vi "Main.vi"() -> ()   [LabVIEW 2020, in "plugin_flodx_ph_probe.lvlib"]
doc: "pH Probe Plugin"
uses:
  plugin_flodx_ph_probe.lvlib
  plugin/process loops/Instrument Manager/loop/Instrument Loop State.ctl
  plugin/process loops/Instrument Manager/connection_info/Connection Info.ctl
  plugin/process loops/Instrument Manager/Instrument State.ctl
  plugin/process loops/UI Manager/Data Display Loop Data.ctl
  plugin/process loops/UI Manager/UI Data.ctl
  plugin/process loops/UI Manager/dialogs/settings/settings.ctl
  <userlib>/RxnRover/PluginCore/src/process loops/Acquisition/Acquisition Config.ctl
  plugin/process loops/Instrument Manager/Instrument Config.ctl
  <userlib>/RxnRover/PluginCore/src/process loops/Logging/loop/Logging Config.ctl
  <userlib>/RxnRover/PluginCore/src/process loops/Logging/log formats/Supported Log File Formats.ctl
  <userlib>/RxnRover/PluginCore/src/process loops/Logging/logger/Logging Start Mode.ctl
  <userlib>/RxnRover/PluginCore/src/process loops/Logging/logger/Logging Stop Mode.ctl
  plugin/process loops/System Control/System Control Data.ctl
  plugin/process loops/UI Manager/UI Display State.ctl
  56943c0d-d29c-4187-abe8-fcc35b9a4d89.vi
  aa3e49f4-ec9d-4bab-88e0-6a79f4e22ab8.vi
  <vilib>/Utility/error.llb/Error Cluster From Error Code.vi
  <vilib>/JDP Science/JSONtext/Variant to JSON Text.vi
  <vilib>/ErrorRing/Error Ring.xnode
  <vilib>/JDP Science/JSONtext/LVClass Serializer/JSONtext LVClass Serializer.lvclass
  <userlib>/RxnRover/PluginCore/src/support/Message Queue/Message Queue.lvlib
  plugin/plugin.lvlib
  <userlib>/RxnRover/PluginCore/src/process loops/Message Queues/Message Queues.lvlib
  <userlib>/RxnRover/PluginCore/src/support/User Event - Stop/User Event - Stop.lvlib
  plugin/process loops/Instrument Manager/Instrument Manager.lvlib
  <userlib>/RxnRover/PluginCore/src/process loops/Logging/Logging.lvlib
  <userlib>/RxnRover/PluginCore/src/process loops/Acquisition/Acquisition.lvlib
  <userlib>/RxnRover/PluginCore/src/process loops/Remote Connection Manager/Remote Connection Manager.lvlib
panel:
  in  "Restart":bool
  out "Comp. Temp(C)":sgl
  out "Address":u8
  in  "Open Calibrate Btn":bool
  out "Logging?":bool
  in  "Time Interval (sec)":i32=1200
  out "Data Graph":cluster{timestamp[], dbl[]}[](graph)
  in  "Open Settings Btn":bool
  in  "Toggle Logging":bool
  out "Measured pH":sgl format="%.2f pH"
  out "VISA resource":refnum<visa-resource-name>
  # "FloDx pH Probe"
  # "Configuration"
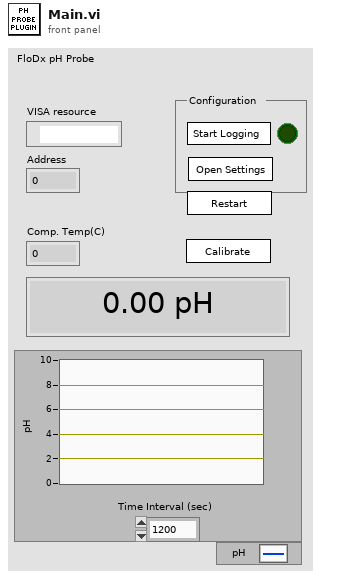
[diagram p1: front panel]
types:
  T1 = typedef "plugin_flodx_ph_probe.lvlib/plugin.lvlib/System Control Data.ctl" = cluster{"Example Value <Replace Me>":dbl, "Log Runs":bool, "Clone":bool}
  T2 = typedef "plugin_flodx_ph_probe.lvlib/plugin.lvlib/UI Data.ctl" = cluster{"UI Controls":cluster{"VISA Resource Ind":refnum<vi>, "Settings Btn":refnum<vi>, "Data Graph":refnum<vi>, "Logging Indicator":refnum<vi>, "Toggle Logging Btn":refnum<vi>, "Measured pH":refnum<vi>, "Temperature (C)":refnum<vi>, "Address":refnum<vi>, "Calibrate Btn":refnum<vi>}, "Plugin Settings":T3}
  T3 = typedef "plugin_flodx_ph_probe.lvlib/plugin.lvlib/settings.ctl" = cluster{"Acquisition Configuration":T4, "Instrument Configuration":T5, "Logging Configuration":T6, "Connection Info":T10}
  T4 = typedef "RxnRover_Plugin_Core.lvlib/Acquisition.lvlib/Acquisition Config.ctl" = cluster{"Query rate (sec)":dbl}
  T5 = typedef "plugin_flodx_ph_probe.lvlib/plugin.lvlib/Instrument Manager.lvlib/Instrument Config.ctl" = cluster{"Address":dbl, "Device":string, "Firmware Version":string}
  T6 = typedef "RxnRover_Plugin_Core.lvlib/Logging.lvlib/Logging Config.ctl" = cluster{"Log Directory":path, "Log File Format":T7, "Log File Name Prefix":string, "Logging Start Mode":T8, "Logging Stop Mode":T9, "Log Interval (Seconds)":dbl}
  T7 = typedef "RxnRover_Plugin_Core.lvlib/Logging.lvlib/Supported Log File Formats.ctl" = enum16{"Spreadsheet (CSV)"}
  T8 = typedef "RxnRover_Plugin_Core.lvlib/Logging.lvlib/Logging Start Mode.ctl" = enum16{"Manual Start", "Log While Running"}
  T9 = typedef "RxnRover_Plugin_Core.lvlib/Logging.lvlib/Logging Stop Mode.ctl" = enum16{"Log Continuously", "Log While Running"}
  T10 = typedef "plugin_flodx_ph_probe.lvlib/plugin.lvlib/Instrument Manager.lvlib/Connection Info.ctl" = cluster{"VISA Resource":refnum<visa-resource-name>, "Address":u8}
  T11 = typedef "plugin_flodx_ph_probe.lvlib/plugin.lvlib/Data Display Loop Data.ctl" = cluster{"Data Timestamps":timestamp[], "Data Values":dbl[], "Previous Run State":bool}
  T12 = typedef "plugin_flodx_ph_probe.lvlib/plugin.lvlib/Instrument Manager.lvlib/Instrument Loop State.ctl" = cluster{"Connection Info":T10, "Running":bool, "Running Since":timestamp, "Instrument State":T13}
  T13 = typedef "plugin_flodx_ph_probe.lvlib/plugin.lvlib/Instrument Manager.lvlib/Instrument State.ctl" = cluster{"pH":sgl, "Temperature (C)":sgl, "Device":string, "Firmware Version":string, "Error Status":bool, "Error Code":i32, "Error Source":string}
  T14 = typedef "RxnRover_Plugin_Core.lvlib/Message Queues.lvlib/All Message Queues.ctl" = cluster{"Acquisition":refnum<queue>, "Instrument":refnum<queue>, "Logging":refnum<queue>, "Remote":refnum<queue>, "System Control":refnum<queue>, "UI":refnum<queue>}
  T15 = typedef "plugin_flodx_ph_probe.lvlib/plugin.lvlib/UI Display State.ctl" = enum16{"Shown", "Hidden"}
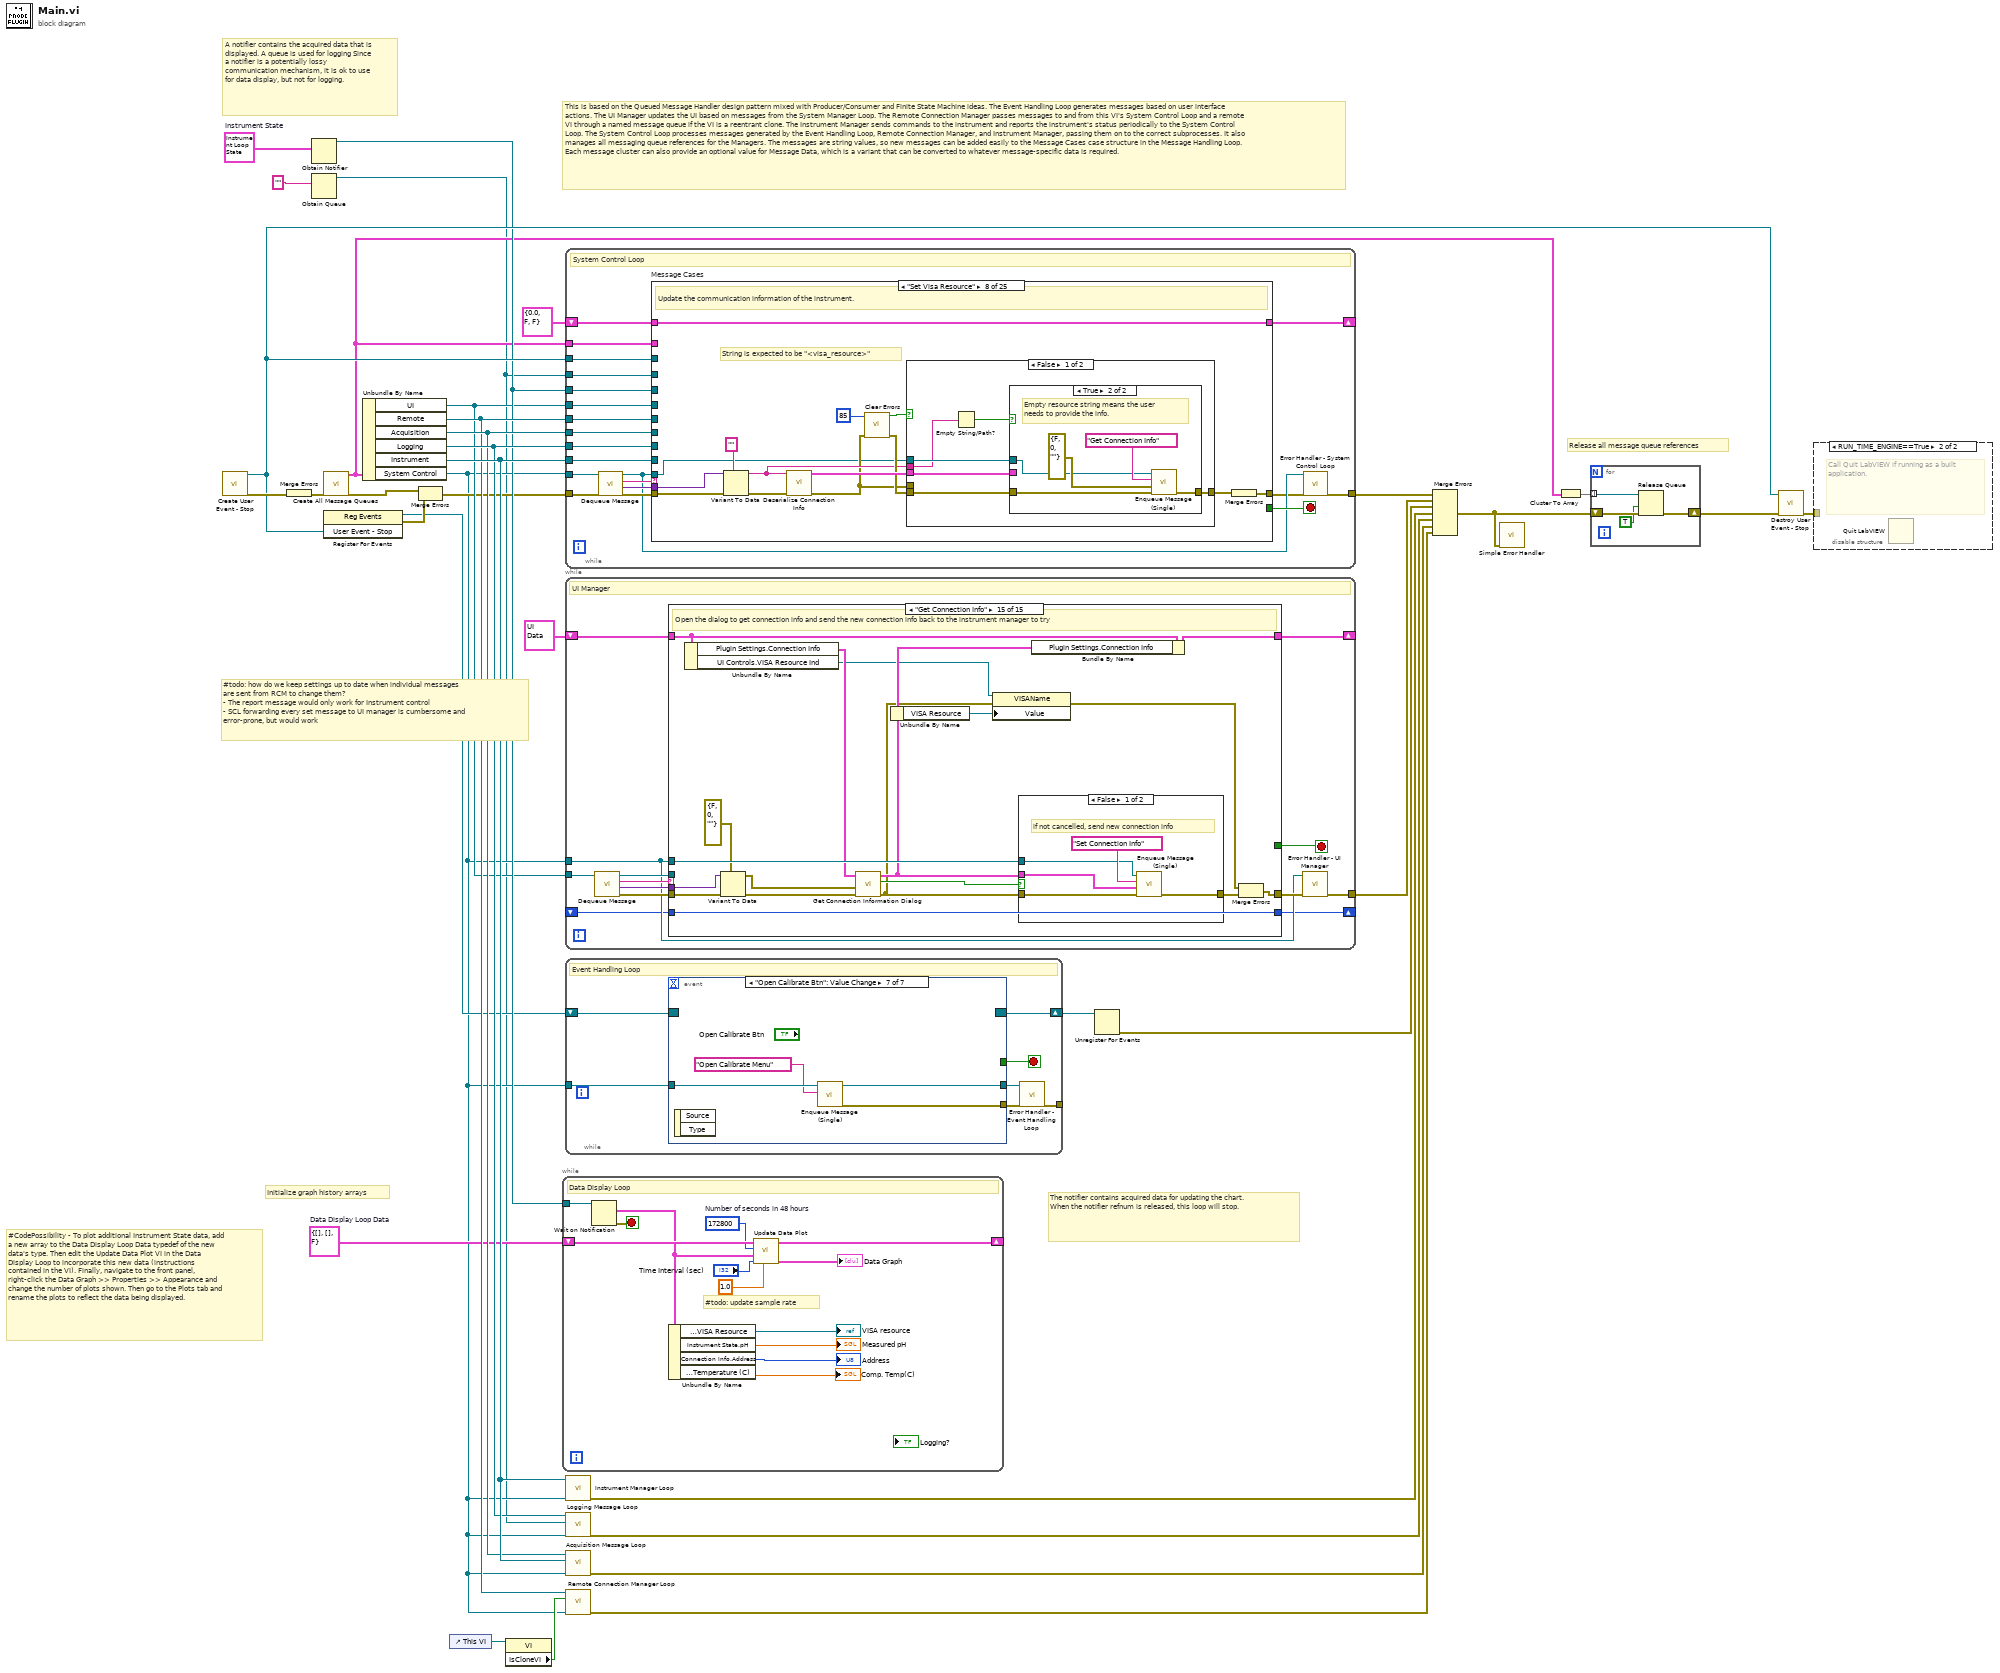
[diagram p0: block diagram]
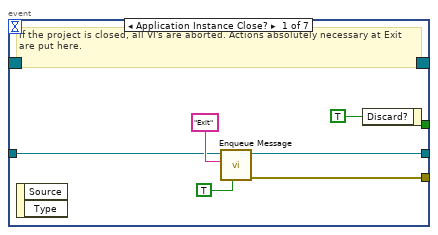
[diagram p2: hidden frame]
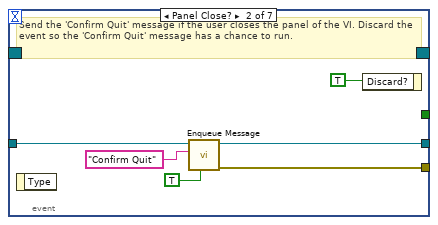
[diagram p3: hidden frame]
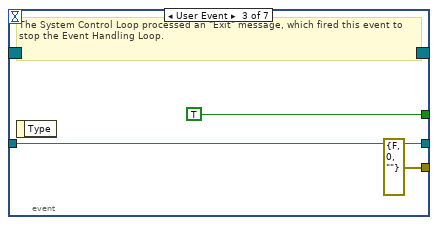
[diagram p4: hidden frame]
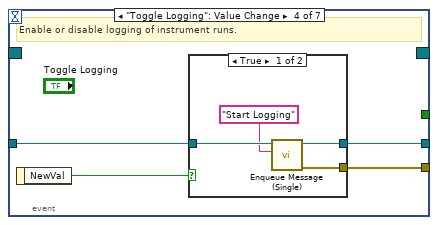
[diagram p5: hidden frame]
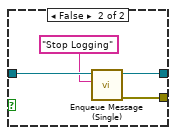
[diagram p6: hidden frame]
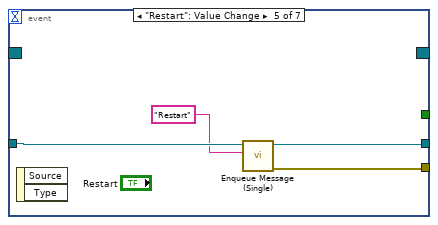
[diagram p7: hidden frame]
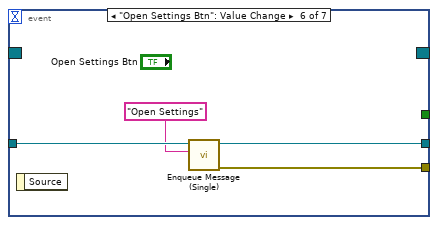
[diagram p8: hidden frame]
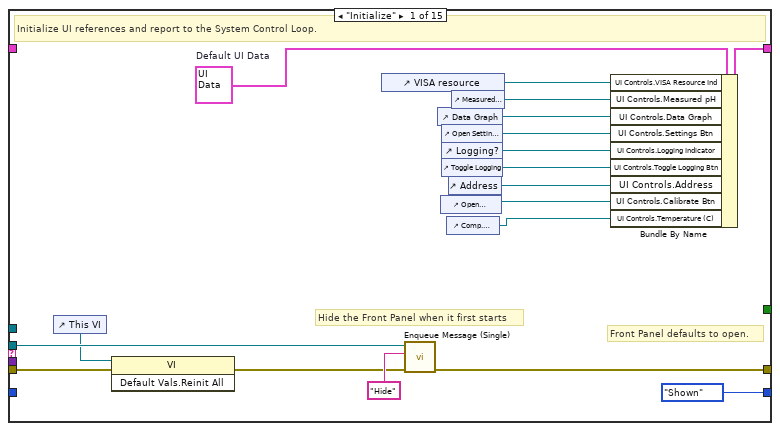
[diagram p9: hidden frame]
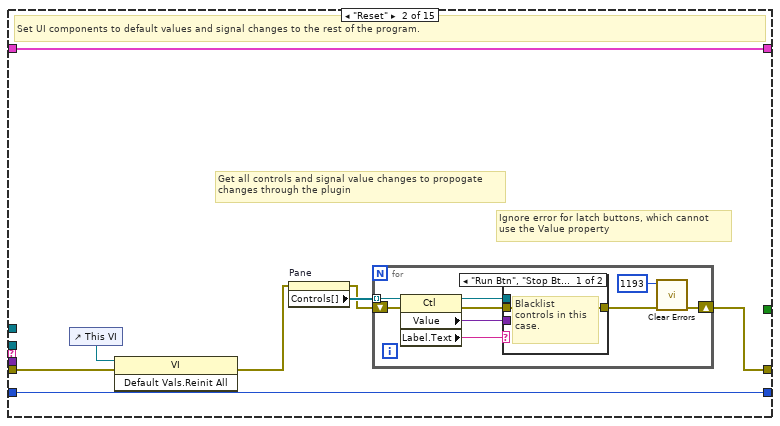
[diagram p10: hidden frame]
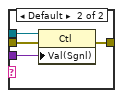
[diagram p11: hidden frame]
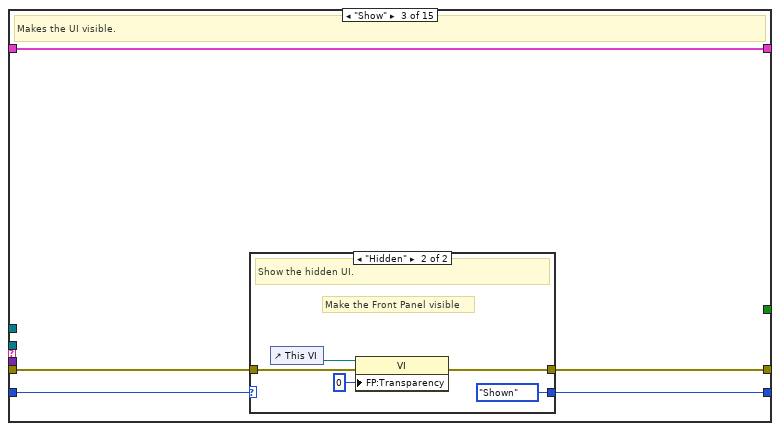
[diagram p12: hidden frame]
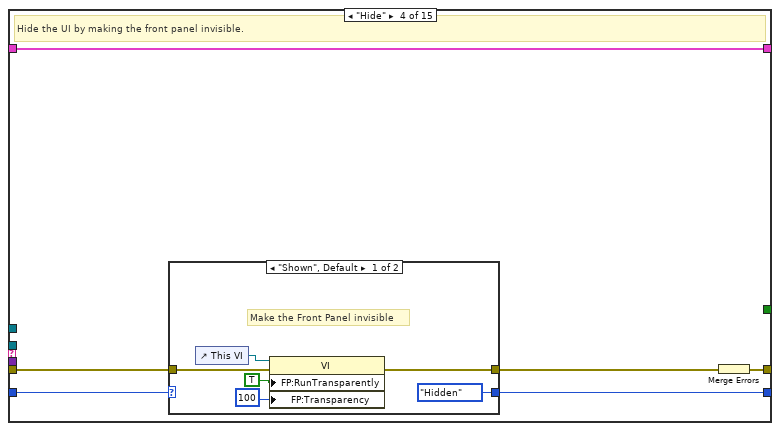
[diagram p14: hidden frame]
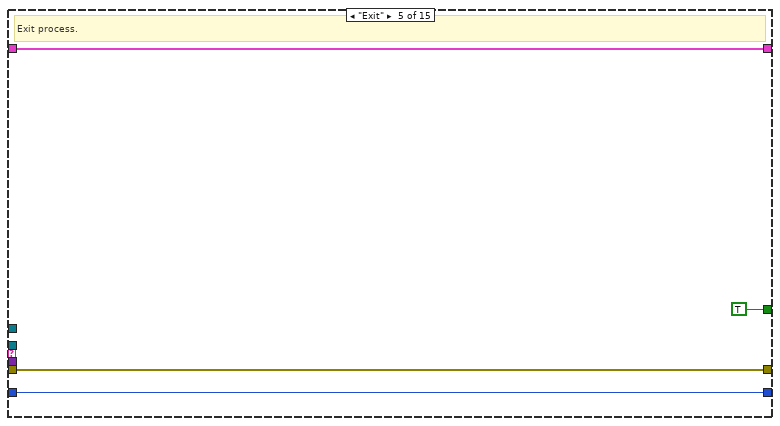
[diagram p16: hidden frame]
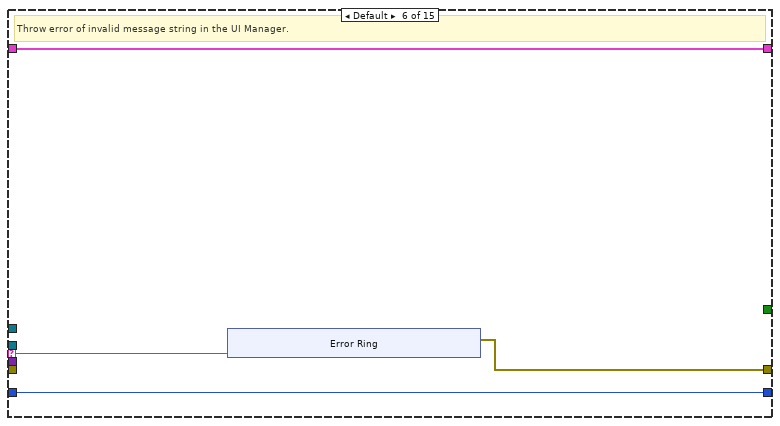
[diagram p17: hidden frame]
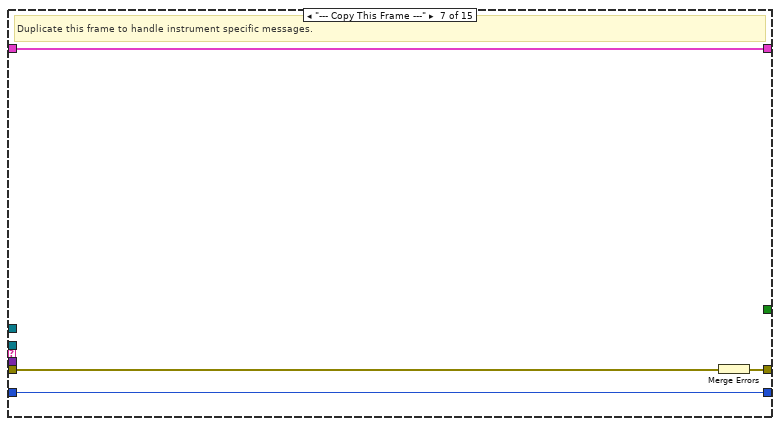
[diagram p18: hidden frame]
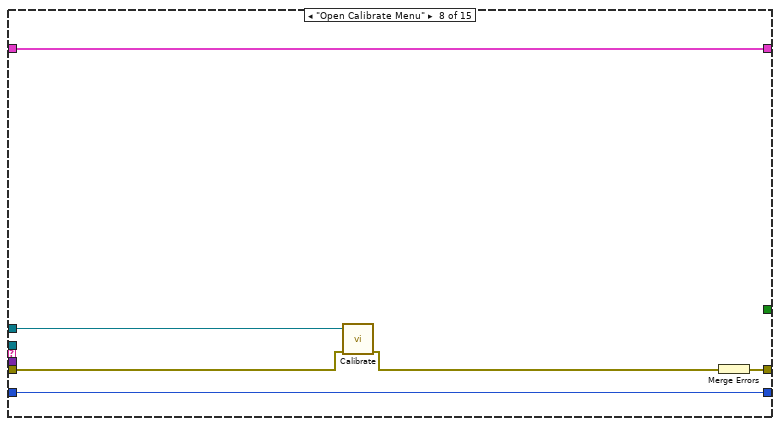
[diagram p19: hidden frame]
diagram:
  w9 = T11 {"Data Timestamps"=[], "Data Values"=[], "Previous Run State"=FALSE}  # Data Display Loop Data
  w12 = T12 {"Connection Info"={"VISA Resource"="", "Address"=0}, "Running"=FALSE, "Running Since"=timestamp(0 s since 1904-01-01), "Instrument State"={"pH"=0.0, "Temperature (C)"=0.0, "Device"="", "Firmware Version"="", "Error Status"=FALSE, "Error Code"=0, "Error Source"=""}}  # Instrument State
  # "#todo: how do we keep settings up to date when individual messages\nare sent from RCM to change them?\n- The report message would only work for Instrument control\n- SCL forwarding every set message to UI manager is cumbersome and\nerror-prone, but would work"
  # "#CodePossibility - To plot additional Instrument State data, add a new array to the Data Display Loop Data typedef of the new data's type. Then edit the Update Data Plot VI in the Data Display Loop to incorporate this new data (instructions contained in the VI). Finally, navigate to the front panel, right-click the Data Graph >> Properties >> Appearance and change the number of plots shown. Then go to the Plots tab and rename the plots to reflect the data being displayed."
  # "Initialize graph history arrays"
  # "A notifier contains the acquired data that is displayed. A queue is used for logging Since a notifier is a potentially lossy communication mechanism, it is ok to use for data display, but not for logging."
  # "The notifier contains acquired data for updating the chart. When the notifier refnum is released, this loop will stop."
  # "Release all message queue references"
  # "This is based on the Queued Message Handler design pattern mixed with Producer/Consumer and Finite State Machine ideas. The Event Handling Loop generates messages based on user interface actions. The UI Manager updates the UI based on messages from the System Manager Loop. The Remote Connection Manager passes messages to and from this VI's System Control Loop and a remote VI through a named message queue if the VI is a reentrant clone. The Instrument Manager sends commands to the instrument and reports the instrument's status periodically to the System Control Loop. The System Control Loop processes messages generated by the Event Handling Loop, Remote Connection Manager, and Instrument Manager, passing them on to the correct subprocesses. It also manages all messaging queue references for the Managers. The messages are string values, so new messages can be added easily to the Message Cases case structure in the Message Handling Loop.  Each message cluster can also provide an optional value for Message Data, which is a variant that can be converted to whatever message-specific data is required."
  n1 = call <userlib>:"Create User Event - Stop.vi"() -> ("error out"=w29:errorcluster, "User Event - Stop"=w25:refnum<user-event>)  [unwired: 10 in]
  n2 = Merge Errors(w29) -> (w28:errorcluster)
  n3 = Obtain Notifier(notification data type=w12) -> (notifier out=w13:refnum<notifier>)  [unwired: 3 in, 2 out]
  n4 = Obtain Queue(element data type="" ("<JSON>")) -> (queue out=w1:refnum<queue>)  [unwired: 4 in, 2 out]
  n5 = call <userlib>:"Create All Message Queues.vi"("error in (no error)"=w28) -> ("error out"=w31:errorcluster, "Message Queues out"=w7:T14)  [unwired: 9 in]
  n6 = register-events(w25) -> (reference out=w10:refnum<event-registration>, error out=w17:errorcluster)  [unwired: 2 in]
  n7 = Unbundle By Name(w7) -> ("UI"=w11:refnum<queue>, "Remote"=w32:refnum<queue>, "Acquisition"=w33:refnum<queue>, "Logging"=w34:refnum<queue>, "Instrument"=w35:refnum<queue>, "System Control"=w4:refnum<queue>)
  n8 = Merge Errors(w31, w17) -> (w5:errorcluster)
  n9 = control-ref of="This VI"() -> (w24:refnum<vi>)
  n10 = property class="VI"(reference=w24) -> ("IsCloneVI"=w23:bool)  [unwired: 1 in, 2 out]
  n11 = while "Data Display Loop" {
    tunnel: w13 -> [w48]
    shift-right: [w45] -> _
    shift-left: w9 -> [w46]
    stop <- w43 stop-if-true
    w40 = 172800  # Number of seconds in 48 hours
    # "#todo: update sample rate"
    # "Data Display Loop"
    n12 = Wait on Notification(notifier=w48) -> (notification=w38:T12, error out=w43:errorcluster)  [unwired: 3 in, 2 out]
    n13 = Unbundle By Name(w38) -> ("Connection Info.VISA Resource"=→"VISA resource":refnum<visa-resource-name>, "Instrument State.pH"=→"Measured pH":sgl, "Connection Info.Address"=→"Address":u8, "Instrument State.Temperature (C)"=→"Comp. Temp(C)":sgl)
    n14 = call "Update Data Plot.vi"("Sample Rate (sec/sample)"=1.0, "Time interval (s)"="Time Interval (sec)", "Instrument State"=w38, "History length (-1; unlimited)"=w40, "Graph History Arrays in"=w46) -> ("Updated Plot History"=→"Data Graph":cluster{timestamp[], dbl[]}[], "Graph History Arrays out"=w45:T11)  [unwired: 5 in]
  }
  n15 = while {
    tunnel: w11 -> [w61]
    tunnel: w4 -> [w52]
    tunnel: [w53] -> w22
    shift-right: [w56] -> _
    shift-left: T2 {"UI Controls"={"VISA Resource Ind"=refnum, "Settings Btn"=refnum, "Data Graph"=refnum, "Logging Indicator"=refnum, "Toggle Logging Btn"=refnum, "Measured pH"=refnum, "Temperature (C)"=refnum, "Address"=refnum, "Calibrate Btn"=refnum}, "Plugin Settings"={"Acquisition Configuration"={"Query rate (sec)"=0.0}, "Instrument Configuration"={"Address"=0.0, "Device"="", "Firmware Version"=""}, "Logging Configuration"={"Log Directory"=path "", "Log File Format"=enum."Spreadsheet (CSV)", "Log File Name Prefix"="", "Logging Start Mode"=enum."Manual Start", "Logging Stop Mode"=enum."Log Continuously", "Log Interval (Seconds)"=0.001}, "Connection Info"={"VISA Resource"="", "Address"=0}}} ("Default UI Data") -> [w55]
    shift-right: [w50] -> _
    shift-left: _ -> [w49]
    stop <- w51 stop-if-true
    # "UI Manager"
    n16 = call <userlib>:"Dequeue Message.vi"("Message Queue"=w61) -> ("error out"=w59:errorcluster, "Message Data"=w57:variant, "Message"=w58:string, "dup Message Queue"=w60:refnum<queue>)  [unwired: 7 in]
    n17 = case shown="\"Get Connection Info\"" w58 {
      selector: w58 -> [_ _ _ _ _ w135 _ _ _ _ _ _ _ w209 _]
      tunnel: w60 -> [w76 _ _ _ _ _ _ _ _ _ _ _ _ _ _]
      tunnel: w59 -> [w70 w83 w105 w117 w131 _ w144 w148 w153 w156 w162 w171 w186 w208 w251]
      tunnel: w57 -> [_ _ _ _ _ _ _ _ _ _ _ _ _ w205 w241]
      tunnel: w52 -> [_ _ _ _ _ _ _ w149 _ _ _ _ w177 _ w246]
      tunnel: [w71 w82 w104 w118 w131 w134 w145 w151 w153 w156 w167 w176 w187 w204 w252] -> w54
      tunnel: [w78 w80 w106 w119 w130 w133 w146 w152 w154 w157 w165 w174 w183 w206 w248] -> w56
      tunnel: w55 -> [_ w80 w106 w119 w130 w133 w146 w152 w154 w157 w165 w174 w184 w203 w249]
      tunnel: [_ _ _ _ TRUE _ _ _ _ _ _ _ _ _ _] -> w51
      tunnel: w49 -> [_ w81 w103 w115 w128 w132 w143 w150 w155 w158 w166 w175 w185 w211 w250]
      tunnel: [UI_Display_State."Shown" ("UI Display State") w81 w102 w114 w128 w132 w143 w150 w155 w158 w166 w175 w185 w211 w250] -> w50
      frame "Initialize" {
        w79 = T2 {"UI Controls"={"VISA Resource Ind"=refnum, "Settings Btn"=refnum, "Data Graph"=refnum, "Logging Indicator"=refnum, "Toggle Logging Btn"=refnum, "Measured pH"=refnum, "Temperature (C)"=refnum, "Address"=refnum, "Calibrate Btn"=refnum}, "Plugin Settings"={"Acquisition Configuration"={"Query rate (sec)"=0.0}, "Instrument Configuration"={"Address"=0.0, "Device"="", "Firmware Version"=""}, "Logging Configuration"={"Log Directory"=path "", "Log File Format"=enum."Spreadsheet (CSV)", "Log File Name Prefix"="", "Logging Start Mode"=enum."Manual Start", "Logging Stop Mode"=enum."Log Continuously", "Log Interval (Seconds)"=0.001}, "Connection Info"={"VISA Resource"="", "Address"=0}}}  # Default UI Data
        # "Front Panel defaults to open."
        # "Hide the Front Panel when it first starts"
        # "Initialize UI references and report to the System Control Loop."
        n18 = control-ref of="This VI"() -> (w72:refnum<vi>)
        n19 = invoke class="VI" method="Default Vals.Reinit All"(reference=w72, error in=w70) -> (error out=w69:errorcluster)  [unwired: 1 in, 2 out]
        n20 = control-ref of="VISA resource"() -> (w77:refnum<vi>)
        n21 = call <userlib>:"Enqueue Message (Single).vi"("error in (no error)"=w69, "Message"="Hide", "Message Queue"=w76) -> ("error out"=w71:errorcluster)  [unwired: 7 in, 1 out]
        n22 = control-ref of="Data Graph"() -> (w65:refnum<vi>)
        n23 = control-ref of="Open Calibrate Btn"() -> (w63:refnum<vi>)
        n24 = control-ref of="Open Settings Btn"() -> (w73:refnum<vi>)
        n25 = control-ref of="Logging?"() -> (w68:refnum<vi>)
        n26 = control-ref of="Toggle Logging"() -> (w67:refnum<vi>)
        n27 = control-ref of="Comp. Temp(C)"() -> (w62:refnum<vi>)
        n28 = control-ref of="Address"() -> (w64:refnum<vi>)
        n29 = control-ref of="Measured pH"() -> (w66:refnum<vi>)
        n30 = Bundle By Name(cluster=w79, "UI Controls.VISA Resource Ind"=w77, "UI Controls.Measured pH"=w66, "UI Controls.Data Graph"=w65, "UI Controls.Settings Btn"=w73, "UI Controls.Logging Indicator"=w68, "UI Controls.Toggle Logging Btn"=w67, "UI Controls.Address"=w64, "UI Controls.Calibrate Btn"=w63, "UI Controls.Temperature (C)"=w62) -> (w78:T2)
      }
      frame "Reset" {
        # "Ignore error for latch buttons, which cannot\nuse the Value property"
        # "Get all controls and signal value changes to propogate\nchanges through the plugin"
        # "Set UI components to default values and signal changes to the rest of the program."
        n31 = control-ref of="This VI"() -> (w87:refnum<vi>)
        n32 = invoke class="VI" method="Default Vals.Reinit All"(reference=w87, error in=w83) -> (error out=w84:errorcluster)  [unwired: 1 in, 2 out]
        n33 = property on="Pane" class="Pane"(error in=w84) -> (error out=w85:errorcluster, "Controls[]"=w86:refnum<vi>[])  [unwired: 1 in, 1 out]
        n34 = for {
          tunnel: w86 -> [w96] mode=indexing
          shift-right: [w90] -> w82
          shift-left: w85 -> [w95]
          n35 = property class="Ctl"(reference=w96, error in=w95) -> (reference out=w94:refnum<vi>, error out=w93:errorcluster, "Value"=w92:variant, "Label.Text"=w88:string)
          n36 = case shown="\"Run Btn\", \"Stop Btn\"" w88 {
            tunnel: w94 -> [_ w101]
            tunnel: w93 -> [w97 w100]
            tunnel: w92 -> [_ w99]
            tunnel: [w97 w98] -> w91
            frame "Run Btn", "Stop Btn" {
              # "Blacklist controls in this case."
            }
            frame Default {
              n37 = property class="Ctl"(reference=w101, error in=w100, "Val(Sgnl)"=w99) -> (error out=w98:errorcluster)  [unwired: 1 out]
            }
          }
          n38 = call <vilib>:"Clear Errors.vi"("error in (no error)"=w91, "specific error code to clear (0: all)"=1193) -> ("error out"=w90:errorcluster)  [unwired: 4 in, 1 out]
        }
      }
      frame "Show" {
        # "Makes the UI visible."
        n39 = case shown="\"Hidden\"" w103 {
          selector: w103 -> [w108 _]
          tunnel: w105 -> [w107 w113]
          tunnel: [w107 w111] -> w104
          tunnel: [w108 UI_Display_State."Shown" ("UI Display State")] -> w102
          frame "Shown", Default {
            # "Do nothing if UI is already shown."
          }
          frame "Hidden" {
            # "Make the Front Panel visible"
            # "Show the hidden UI."
            n40 = control-ref of="This VI"() -> (w112:refnum<vi>)
            n41 = property class="VI"(reference=w112, error in=w113, "FP:Transparency"=u8 0 ("Front Panel Window:Transparency")) -> (error out=w111:errorcluster)  [unwired: 1 out]
          }
        }
      }
      frame "Hide" {
        # "Hide the UI by making the front panel invisible."
        n42 = case shown="\"Shown\", Default" w115 {
          selector: w115 -> [_ w127]
          tunnel: w117 -> [w122 w126]
          tunnel: [w121 w126] -> w116
          tunnel: [UI_Display_State."Hidden" ("UI Display State") w127] -> w114
          frame "Shown", Default {
            # "Make the Front Panel invisible"
            n43 = control-ref of="This VI"() -> (w125:refnum<vi>)
            n44 = property class="VI"(reference=w125, error in=w122, "FP:RunTransparently"=TRUE ("Front Panel Window:Run VI Transparently"), "FP:Transparency"=u8 100 ("Front Panel Window:Transparency")) -> (error out=w121:errorcluster)  [unwired: 1 out]
          }
          frame "Hidden" {
          }
        }
        n45 = Merge Errors(w116) -> (w118:errorcluster)
      }
      frame "Exit" {
        # "Exit process."
      }
      frame Default {
        # "Throw error of invalid message string in the UI Manager."
        n46 = xnode "Error Ring"("parameter 0"=w135) -> ("error out"=w134:errorcluster)
      }
      frame "--- Copy This Frame ---" {
        # "Duplicate this frame to handle instrument specific messages."
        n47 = Merge Errors(w144) -> (w145:errorcluster)
      }
      frame "Open Calibrate Menu" {
        n48 = call "Calibrate.vi"("error in (no error)"=w148, "Message Queue"=w149) -> ("error out"=w147:errorcluster)  [unwired: 9 in]
        n49 = Merge Errors(w147) -> (w151:errorcluster)
      }
      frame "Instrument Started" {
        # "The instrument started. Ensure that the UI reflects this."
      }
      frame "Instrument Stopped" {
        # "The instrument stopped. Ensure that the UI reflects this."
      }
      frame "Logging Started" {
        w159 = TRUE  # Logging is on
        # "Indicate that logging started."
        n50 = Unbundle By Name(w165) -> ("UI Controls.Logging Indicator"=w164:refnum<vi>, "UI Controls.Toggle Logging Btn"=w163:refnum<vi>)
        n51 = property class="Bool (strict)"(reference=w164, error in=w162, "Value"=w159) -> (error out=w161:errorcluster)  [unwired: 1 out]
        n52 = property class="Bool"(reference=w163, error in=w162, "Value"=w159) -> (error out=w160:errorcluster)  [unwired: 1 out]
        n53 = Merge Errors(w161, w160) -> (w167:errorcluster)
      }
      frame "Logging Stopped" {
        w168 = FALSE  # Logging is off
        # "Indicate that logging stopped."
        n54 = Unbundle By Name(w174) -> ("UI Controls.Logging Indicator"=w173:refnum<vi>, "UI Controls.Toggle Logging Btn"=w172:refnum<vi>)
        n55 = property class="Bool (strict)"(reference=w173, error in=w171, "Value"=w168) -> (error out=w170:errorcluster)  [unwired: 1 out]
        n56 = property class="Bool"(reference=w172, error in=w171, "Value"=w168) -> (error out=w169:errorcluster)  [unwired: 1 out]
        n57 = Merge Errors(w170, w169) -> (w176:errorcluster)
      }
      frame "Open Settings" {
        # "Open the settings dialog and send new settings to other loops"
        n58 = Unbundle By Name(w184) -> ("Plugin Settings"=w182:T3)
        n59 = call "Settings Dialog.vi"("error in (no error)"=w186, "System Control Queue"=w177, "Plugin Settings"=w182) -> ("error out"=w181:errorcluster, "Cancelled?"=w179:bool, "Plugin Settings out"=w178:T3)  [unwired: 6 in]
        n60 = case shown="False" w179 {
          tunnel: w181 -> [w193 w201]
          tunnel: [w200 w201] -> w180
          tunnel: w178 -> [w195 _]
          tunnel: w177 -> [w194 _]
          frame False {
            # "Settings dialog was not cancelled, send new settings"
            n61 = Unbundle By Name(w195) -> ("Acquisition Configuration"=w198:T4)
            n62 = Unbundle By Name(w195) -> ("Instrument Configuration"=w196:T5)
            n63 = Unbundle By Name(w195) -> ("Logging Configuration"=w191:T6)
            n64 = call <userlib>:"Enqueue Message (Single).vi"("error in (no error)"=w193, "Message Data"=w198, "Message"="New Acquisition Config", "Message Queue"=w194) -> ("error out"=w188:errorcluster)  [unwired: 6 in, 1 out]
            n65 = call <userlib>:"Enqueue Message (Single).vi"("error in (no error)"=w193, "Message Data"=w196, "Message"="New Instrument Config", "Message Queue"=w194) -> ("error out"=w189:errorcluster)  [unwired: 6 in, 1 out]
            n66 = call <userlib>:"Enqueue Message (Single).vi"("error in (no error)"=w193, "Message Data"=w191, "Message"="New Logging Config", "Message Queue"=w194) -> ("error out"=w190:errorcluster)  [unwired: 6 in, 1 out]
            n67 = Merge Errors(w188, w189, w190) -> (w200:errorcluster)
          }
          frame True {
            # "The settings dialog was cancelled, don't send anything"
          }
        }
        n68 = Bundle By Name(cluster=w184, "Plugin Settings"=w178) -> (w183:T2)
        n69 = Merge Errors(w180) -> (w187:errorcluster)
      }
      frame "Acquisition Config", "Instrument Config", "Logging Config" {
        # "Store the settings provided by another loop to display to the user"
        n70 = Scan From String(format string="%s Config", input string=w209, error in=w208) -> (error out=w202:errorcluster, output 1=w207:string)  [unwired: 2 in, 2 out]
        n71 = case shown="\"Acquisition\"" w207 {
          tunnel: w203 -> [w213 w220 w227 w234]
          tunnel: [w213 w219 w226 w233] -> w206
          tunnel: w205 -> [_ w218 w225 w231]
          tunnel: w202 -> [w212 w217 w224 w230]
          tunnel: [w212 w216 w221 w229] -> w204
          frame Default {
            # "I don't know how we would get here, but do nothing\nif an invalid string is given."
          }
          frame "Acquisition" {
            n72 = Variant To Data(error in=w217, type=T4 {"Query rate (sec)"=1.0} ("Acquisition Configuration"), Variant=w218) -> (data=w215:T4, error out=w216:errorcluster)
            n73 = Bundle By Name(cluster=w220, "Plugin Settings.Acquisition Configuration"=w215) -> (w219:T2)
          }
          frame "Instrument" {
            n74 = Variant To Data(error in=w224, type=T5 {"Address"=0.0, "Device"="", "Firmware Version"=""} ("Instrument Configuration"), Variant=w225) -> (data=w222:T5, error out=w221:errorcluster)
            n75 = Bundle By Name(cluster=w227, "Plugin Settings.Instrument Configuration"=w222) -> (w226:T2)
          }
          frame "Logging" {
            n76 = Variant To Data(error in=w230, type=T6 {"Log Directory"=path "", "Log File Format"=enum."Spreadsheet (CSV)", "Log File Name Prefix"="experiment_", "Logging Start Mode"=enum."Manual Start", "Logging Stop Mode"=enum."Log Continuously", "Log Interval (Seconds)"=0.001} ("Logging Configuration"), Variant=w231) -> (data=w228:T6, error out=w229:errorcluster)
            n77 = Bundle By Name(cluster=w234, "Plugin Settings.Logging Configuration"=w228) -> (w233:T2)
          }
        }
      }
      frame "Get Connection Info" {
        # "Open the dialog to get connection info and send the new connection info back to the instrument manager to try"
        n78 = Unbundle By Name(w249) -> ("Plugin Settings.Connection Info"=w245:T10, "UI Controls.VISA Resource Ind"=w238:refnum<vi>)
        n79 = Variant To Data(error in=w251, type=errorcluster {"status"=FALSE, "code"=0, "source"=""} ("error out"), Variant=w241) -> (data=w240:errorcluster, error out=w243:errorcluster)
        n80 = call "Get Connection Information Dialog.vi"("error in (no error)"=w243, "previous attempt error (no error)"=w240, "Connection Info"=w245) -> ("error out"=w236:errorcluster, "Cancelled?"=w244:bool, "Connection Info out"=w239:T10)  [unwired: 6 in]
        n81 = Unbundle By Name(w239) -> ("VISA Resource"=w237:refnum<visa-resource-name>)
        n82 = property class="VISAName"(reference=w238, error in=w236, "Value"=w237) -> (error out=w235:errorcluster)  [unwired: 1 out]
        n83 = case shown="False" w244 {
          tunnel: w236 -> [w254 w262]
          tunnel: [w257 w261] -> w247
          tunnel: w239 -> [w253 _]
          tunnel: w246 -> [w255 w259]
          frame False {
            # "if not cancelled, send new connection info"
            n84 = call <userlib>:"Enqueue Message (Single).vi"("error in (no error)"=w254, "Message Data"=w253, "Message"="Set Connection Info", "Message Queue"=w255) -> ("error out"=w257:errorcluster)  [unwired: 6 in, 1 out]
          }
          frame True {
            # "If the user cancels the connection,\nclose the plugin."
            n85 = call <userlib>:"Enqueue Message (Single).vi"("Priority Message? (F)"=TRUE, "error in (no error)"=w262, "Message"="Exit", "Message Queue"=w259) -> ("error out"=w261:errorcluster)  [unwired: 6 in, 1 out]
          }
        }
        n86 = Bundle By Name(cluster=w249, "Plugin Settings.Connection Info"=w239) -> (w248:T2)
        n87 = Merge Errors(w235, w247) -> (w252:errorcluster)
      }
    }
    n88 = call "Error Handler - UI Manager.vi"("error in (no error)"=w54, "Message Queue"=w52) -> ("dup error in"=w53:errorcluster)  [unwired: 8 in, 1 out]
  }
  n89 = while {
    tunnel: w4 -> [w269]
    shift-right: [w267] -> w26
    shift-left: w10 -> [w268]
    tunnel: [w263] -> _
    stop <- w265 stop-if-true
    # "Event Handling Loop"
    n90 = event shown="[6] \"Open Calibrate Btn\": Value Change" {
      selector: w268 -> [_ _ _ _ _ _ _]
      dyn-events: [_ _ _ _ _ _ _] -> w267
      timeout: _ -> [_ _ _ _ _ _ _]
      tunnel: [_ _ TRUE ("Discard?") _ _ _ _] -> w265
      tunnel: w269 -> [w272 w280 w284 w288 w300 w304 w306]
      tunnel: [w270 w279 errorcluster {"status"=FALSE, "code"=0, "source"=""} ("error out") w285 w298 w301 w308] -> w266
      tunnel: [w271 w278 w284 w287 w299 w303 w307] -> w264
      event Application Instance Close? {
        # "If the project is closed, all VI's are aborted. Actions absolutely necessary at Exit are put here."
        n91 = event-data() -> ()  [unwired: 1 in, 2 out]
        n92 = call-poly <userlib>:"Enqueue Message.vi"("Priority Message? (F)"=TRUE, "Message"="Exit", "Message Queue"=w272) -> ("error out"=w270:errorcluster, "dup Message Queue"=w271:refnum<queue>)  [unwired: 7 in]
        n93 = event-data("Discard?"=TRUE) -> ()  [unwired: 1 in, 1 out]
      }
      event Panel Close? {
        # "Send the 'Confirm Quit' message if the user closes the panel of the VI. Discard the event so the 'Confirm Quit' message has a chance to run."
        n94 = event-data() -> ()  [unwired: 1 in, 1 out]
        n95 = call-poly <userlib>:"Enqueue Message.vi"("Priority Message? (F)"=TRUE, "Message"="Confirm Quit", "Message Queue"=w280) -> ("error out"=w279:errorcluster, "dup Message Queue"=w278:refnum<queue>)  [unwired: 7 in]
        n96 = event-data("Discard?"=TRUE) -> ()  [unwired: 1 in, 1 out]
      }
      event User Event {
        # "The System Control Loop processed an \"Exit\" message, which fired this event to stop the Event Handling Loop."
        n97 = event-data() -> ()  [unwired: 1 in, 1 out]
      }
      event "Toggle Logging": Value Change {
        # "Enable or disable logging of instrument runs."
        n98 = event-data() -> ("NewVal"=w286:bool)  [unwired: 1 in]
        n99 = case shown="True" w286 {
          tunnel: w288 -> [w292 w296]
          tunnel: [w291 w295] -> w287
          tunnel: [w289 w293] -> w285
          frame True {
            n100 = call <userlib>:"Enqueue Message (Single).vi"("Message"="Start Logging", "Message Queue"=w292) -> ("error out"=w289:errorcluster, "dup Message Queue"=w291:refnum<queue>)  [unwired: 8 in]
          }
          frame False {
            n101 = call <userlib>:"Enqueue Message (Single).vi"("Message"="Stop Logging", "Message Queue"=w296) -> ("error out"=w293:errorcluster, "dup Message Queue"=w295:refnum<queue>)  [unwired: 8 in]
          }
        }
      }
      event "Restart": Value Change {
        n102 = event-data() -> ()  [unwired: 1 in, 2 out]
        n103 = call <userlib>:"Enqueue Message (Single).vi"("Message"="Restart", "Message Queue"=w300) -> ("error out"=w298:errorcluster, "dup Message Queue"=w299:refnum<queue>)  [unwired: 8 in]
      }
      event "Open Settings Btn": Value Change {
        n104 = event-data() -> ()  [unwired: 1 in, 1 out]
        n105 = call <userlib>:"Enqueue Message (Single).vi"("Message"="Open Settings", "Message Queue"=w304) -> ("error out"=w301:errorcluster, "dup Message Queue"=w303:refnum<queue>)  [unwired: 8 in]
      }
      event "Open Calibrate Btn": Value Change {
        n106 = event-data() -> ()  [unwired: 1 in, 2 out]
        n107 = call <userlib>:"Enqueue Message (Single).vi"("Message"="Open Calibrate Menu", "Message Queue"=w306) -> ("error out"=w308:errorcluster, "dup Message Queue"=w307:refnum<queue>)  [unwired: 8 in]
      }
    }
    n108 = call "Error Handler - Event Handling Loop.vi"("error in (no error)"=w266, "Message Queue"=w264) -> ("dup error in"=w263:errorcluster)  [unwired: 8 in, 1 out]
  }
  n109 = while {
    tunnel: w4 -> [w320]
    shift-right: [w327] -> _
    shift-left: T1 {"Example Value <Replace Me>"=0.0, "Log Runs"=FALSE, "Clone"=FALSE} ("Default Data") -> [w328]
    tunnel: w25 -> [w325]
    tunnel: w5 -> [w324]
    tunnel: [w318] -> w30
    tunnel: w35 -> [w316]
    tunnel: w32 -> [w315]
    tunnel: w11 -> [w314]
    tunnel: w33 -> [w313]
    tunnel: w34 -> [w312]
    tunnel: w13 -> [w311]
    tunnel: w1 -> [w310]
    tunnel: w7 -> [w309]
    stop <- w326 stop-if-true
    # "System Control Loop"
    n110 = call <userlib>:"Dequeue Message.vi"("error in (no error)"=w324, "Message Queue"=w320) -> ("error out"=w323:errorcluster, "Message Data"=w321:variant, "Message"=w322:string, "dup Message Queue"=w319:refnum<queue>)  [unwired: 6 in]
    n111 = case "Message Cases" shown="\"Set Visa Resource\"" w322 {
      selector: w322 -> [_ _ _ w370 w383 w394 w412 _ w462 w469 w476 _ w515 w525 w532 w539 w552 w557 w565 w574 w588 w599 w610 w635 _]
      tunnel: w319 -> [w329 _ w350 _ _ _ _ w425 _ _ _ _ _ _ _ _ _ _ _ _ _ _ _ _ _]
      tunnel: w323 -> [w332 w347 w354 _ _ w397 w415 w430 w465 w472 w484 w512 w517 w528 w535 w542 w554 w561 w568 w577 w592 w602 _ w629 w637]
      tunnel: [w331 w341 w352 w373 w384 w403 w417 w427 w466 w473 w490 w511 w522 w529 w536 w543 w555 w562 w569 w578 w590 w603 w609 w627 w637] -> w317
      tunnel: w328 -> [_ w346 w353 w369 w385 w404 w418 w438 w464 w471 w489 w513 w523 w530 w537 w544 w556 w563 w570 w579 w591 w604 w608 w633 w638]
      tunnel: [w333 w346 w353 w369 w385 w404 w418 w438 w464 w471 w489 w513 w523 w530 w537 w544 w556 w563 w570 w579 w591 w604 w608 w633 w638] -> w327
      tunnel: [_ _ _ TRUE _ _ _ _ _ _ _ _ _ _ _ _ _ _ _ _ _ _ _ _ _] -> w326
      tunnel: w321 -> [_ w345 _ w374 _ w393 w411 w429 w461 w468 w477 w508 _ w526 w533 w540 w550 w558 w566 w575 w587 w600 w611 w623 _]
      tunnel: w325 -> [_ _ _ w371 _ _ _ _ _ _ _ _ _ _ _ _ _ _ _ _ _ _ _ _ _]
      tunnel: w316 -> [_ _ _ w366 _ w398 _ _ _ w467 _ _ _ _ _ _ _ _ _ _ _ w598 _ _ _]
      tunnel: w315 -> [_ _ _ w365 _ w401 w416 _ _ _ w494 _ _ _ _ _ _ _ _ w573 _ _ w612 _ _]
      tunnel: w314 -> [_ _ _ w364 _ w400 _ _ w460 _ w493 w510 _ w524 w531 w538 _ _ _ w572 _ _ w605 _ _]
      tunnel: w313 -> [_ _ _ w368 _ w402 _ _ _ _ w495 _ _ _ _ _ _ _ w564 _ w586 _ w607 _ _]
      tunnel: w312 -> [_ _ _ w367 _ w399 _ _ _ _ w486 _ w520 _ _ _ _ w559 _ _ _ _ w606 _ _]
      tunnel: w311 -> [_ _ _ w361 _ _ _ _ _ _ _ _ _ _ _ _ _ _ _ _ _ _ _ w632 _]
      tunnel: w310 -> [_ _ _ w359 _ _ _ _ _ _ _ _ _ _ _ _ _ _ _ _ _ _ _ w630 _]
      tunnel: w309 -> [_ _ _ _ _ _ _ _ _ _ _ _ _ _ _ _ w545 _ _ _ _ _ _ w624 _]
      frame "Initialize" {
        w334 = T1 {"Example Value <Replace Me>"=0.0, "Log Runs"=FALSE, "Clone"=FALSE}  # Default Data
        # "Initialize the system control loop and system."
        n112 = control-ref of="This VI"() -> ()  [unwired: 1 out]
        n113 = property on="Property Node" class="VI"() -> ("IsCloneVI"=w330:bool)  [unwired: 2 in, 2 out]
        n114 = Bundle By Name(cluster=w334, "Clone"=w330) -> (w333:T1)
        n115 = case shown="False" w330 {
          tunnel: w332 -> [w338 w340]
          tunnel: [w337 w340] -> w331
          tunnel: w329 -> [w336 _]
          frame False {
            # "Ask the user for connection info if this isn't a reentrant clone"
            n116 = call <userlib>:"Enqueue Message (Single).vi"("error in (no error)"=w338, "Message Data"=errorcluster {"status"=FALSE, "code"=0, "source"=""} ("error out"), "Message"="Get Connection Info", "Message Queue"=w336) -> ("error out"=w337:errorcluster)  [unwired: 6 in, 1 out]
          }
          frame True {
            # "Reentrant clone. It is the responsibility of the RCM to send the connection info command."
          }
        }
      }
      frame "Error" {
        # "#CodeRecommended - If you ever change the name of this \"Error\" message, you'll need to update the name in the Check Loop Error.vi as well."
        # "#CodeRecommended - Consider creating a system for logging errors in some way. These errors are for notification purposes only. Handling of specific errors should be performed in the message frames that generated the error."
        # "Error - Display an error dialog. This message is sent by the \"Error Handler\" VIs at the end of other loops in this application."
        n117 = Variant To Data(error in=w347, type=errorcluster {"status"=FALSE, "code"=0, "source"=""} ("error constant"), Variant=w345) -> (data=w343:errorcluster, error out=w342:errorcluster)
        n118 = call <vilib>:"Simple Error Handler.vi"("error in (no error)"=w343) -> ()  [unwired: 4 in, 5 out]
        n119 = Merge Errors(w342) -> (w341:errorcluster)
      }
      frame "Confirm Quit" {
        # "#CodeNeeded - If you want to provide an \"Are you sure\" dialog (or some other notification) before the application exits, place that code here. This message is typically sent from a Panel Close? event."
        # "Confirm Quit - Message that can confirm whether or not the user wants to exit the application."
        n120 = call-poly <userlib>:"Enqueue Message.vi"("Priority Message? (F)"=TRUE, "error in (no error)"=w354, "Message"="Exit", "Message Queue"=w350) -> ("error out"=w351:errorcluster)  [unwired: 6 in, 1 out]
        n121 = Merge Errors(w351) -> (w352:errorcluster)
      }
      frame "Exit" {
        # "Order other processes to exit"
        # "Begin the application closing procedure by sending \"Exit\" commands to all running processes."
        n122 = Variant To Data(type=errorcluster {"status"=FALSE, "code"=0, "source"=""} ("error constant"), Variant=w374) -> (data=w375:errorcluster)  [unwired: 1 in, 1 out]
        n123 = Build Array(w364, w365, w368, w367, w366) -> (w363:refnum<queue>[])
        n124 = call <vilib>:"Clear Errors.vi"("error in (no error)"=w375, "specific error code to clear (0: all)"=5000) -> ("error out"=w356:errorcluster)  [unwired: 4 in, 1 out]
        n125 = call <vilib>:"Simple Error Handler.vi"("error in (no error)"=w356) -> ()  [unwired: 4 in, 5 out]
        n126 = for {
          tunnel: w370 -> [w381]
          tunnel: w363 -> [w380] mode=indexing
          shift-right: [w379] -> w372
          shift-left: _ -> [w378]
          n127 = call <userlib>:"Enqueue Message (Single).vi"("Priority Message? (F)"=TRUE, "Message"=w381, "Message Queue"=w380) -> ("error out"=w382:errorcluster)  [unwired: 7 in, 1 out]
          n128 = Merge Errors(w382, w378) -> (w379:errorcluster)
        }
        n129 = Release Notifier(notifier=w361) -> (error out=w360:errorcluster)  [unwired: 2 in, 2 out]
        n130 = Release Queue(queue=w359) -> (error out=w357:errorcluster)  [unwired: 2 in, 2 out]
        n131 = call <userlib>:"Fire User Event - Stop.vi"("User Event - Stop"=w371) -> ("error out"=w358:errorcluster)  [unwired: 10 in]
        n132 = Merge Errors(w358, w357, w360, w372) -> (w373:errorcluster)
      }
      frame Default {
        # "'Default' case only runs if there is a message that isn't defined in any of the other cases.  Output a programming error."
        n133 = xnode "Error Ring"("parameter 0"=w383) -> ("error out"=w384:errorcluster)
      }
      frame "---Copy This Frame---" {
        # "Sends the message to each process in the array."
        # "#CodeRecommended - Change connections to build an array of the processes that will receive this message"
        # "Duplicate this frame when creating new messages.  Change this comment in the duplicated frame to describe this message."
        n134 = Build Array(w400, w401, w402, w399, w398) -> (w395:refnum<queue>[])
        n135 = for {
          tunnel: w395 -> [w408] mode=indexing
          tunnel: w394 -> [w410]
          tunnel: w393 -> [w409]
          shift-right: [w407] -> w396
          shift-left: w397 -> [w405]
          n136 = call <userlib>:"Enqueue Message (Single).vi"("Message Data"=w409, "Message"=w410, "Message Queue"=w408) -> ("error out"=w406:errorcluster)  [unwired: 7 in, 1 out]
          n137 = Merge Errors(w406, w405) -> (w407:errorcluster)
        }
        n138 = Merge Errors(w396) -> (w403:errorcluster)
      }
      frame "Set Remote Queue" {
        # "Sends the message to each process in the array."
        # "Bounce this message back to the Remote Control Manager to set the remote queue to publish messages to."
        n139 = Build Array(w416) -> (w413:refnum<queue>[])
        n140 = for {
          tunnel: w413 -> [w422] mode=indexing
          tunnel: w412 -> [w424]
          tunnel: w411 -> [w423]
          shift-right: [w421] -> w414
          shift-left: w415 -> [w419]
          n141 = call <userlib>:"Enqueue Message (Single).vi"("Message Data"=w423, "Message"=w424, "Message Queue"=w422) -> ("error out"=w420:errorcluster)  [unwired: 7 in, 1 out]
          n142 = Merge Errors(w420, w419) -> (w421:errorcluster)
        }
        n143 = Merge Errors(w414) -> (w417:errorcluster)
      }
      frame "Set Visa Resource" {
        # "String is expected to be \"<visa_resource>\""
        # "Update the communication information of the instrument."
        n144 = Variant To Data(error in=w430, type="", Variant=w429) -> (data=w432:string, error out=w437:errorcluster)
        n145 = call "Deserialize Connection Info.vi"("error in (no error)"=w437, "Connection Info String"=w432) -> ("error out"=w431:errorcluster, "Deserialized Connection Info"=w436:T10)  [unwired: 8 in]
        n146 = call <vilib>:"Clear Errors.vi"("error in (no error)"=w431, "specific error code to clear (0: all)"=85) -> ("error out"=w434:errorcluster, "specific error cleared?"=w433:bool)  [unwired: 4 in]
        n147 = case shown="False" w433 {
          tunnel: w425 -> [w444 w458]
          tunnel: w436 -> [w443 _]
          tunnel: [w439 w456] -> w428
          tunnel: w434 -> [w442 w457]
          tunnel: w432 -> [w440 _]
          tunnel: w431 -> [_ w455]
          frame False {
            n148 = Empty String/Path?(string/path=w440) -> (empty?=w441:bool)
            n149 = case shown="True" w441 {
              tunnel: w444 -> [w448 w450]
              tunnel: w443 -> [w447 _]
              tunnel: [w445 w451] -> w439
              tunnel: w442 -> [w446 w452]
              frame False {
                n150 = call <userlib>:"Enqueue Message (Single).vi"("error in (no error)"=w446, "Message Data"=w447, "Message"="Set Connection Info", "Message Queue"=w448) -> ("error out"=w445:errorcluster)  [unwired: 6 in, 1 out]
              }
              frame True {
                # "Empty resource string means the user needs to provide the info."
                n151 = call <userlib>:"Enqueue Message (Single).vi"("error in (no error)"=w452, "Message Data"=errorcluster {"status"=FALSE, "code"=0, "source"=""} ("error out"), "Message"="Get Connection Info", "Message Queue"=w450) -> ("error out"=w451:errorcluster)  [unwired: 6 in, 1 out]
              }
            }
          }
          frame True {
            # "If error 85 occurred, then the connection info string was invalid because the Scan from String function failed. The error being returned should report the exact issue."
            n152 = call <userlib>:"Enqueue Message (Single).vi"("error in (no error)"=w457, "Message Data"=w455, "Message"="Invalid Connection Info", "Message Queue"=w458) -> ("error out"=w456:errorcluster)  [unwired: 6 in, 1 out]
          }
        }
        n153 = Merge Errors(w428) -> (w427:errorcluster)
      }
      frame "Get Connection Info" {
        # "Request connection information from the user."
        n154 = call <userlib>:"Enqueue Message (Single).vi"("error in (no error)"=w465, "Message Data"=w461, "Message"=w462, "Message Queue"=w460) -> ("error out"=w463:errorcluster)  [unwired: 6 in, 1 out]
        n155 = Merge Errors(w463) -> (w466:errorcluster)
      }
      frame "Set Connection Info" {
        # "Request connection information from the user."
        n156 = call <userlib>:"Enqueue Message (Single).vi"("error in (no error)"=w472, "Message Data"=w468, "Message"=w469, "Message Queue"=w467) -> ("error out"=w470:errorcluster)  [unwired: 6 in, 1 out]
        n157 = Merge Errors(w470) -> (w473:errorcluster)
      }
      frame "Valid Connection Info" {
        # "Convert before sending"
        # "When a Valid Communication Info has been chosen, start the other processes."
        n158 = Unbundle By Name(w489) -> ("Log Runs"=w488:bool)
        n159 = call "To JSON Text.vim"("error in (no error)"=w484, "Anything"=w477) -> ("error out"=w483:errorcluster, "<JSON>"=w482:string)  [unwired: 8 in]
        n160 = call <userlib>:"Enqueue Message (Single).vi"("error in (no error)"=w483, "Message Data"=w482, "Message"=w476, "Message Queue"=w486) -> ("error out"=w487:errorcluster, "dup Message Queue"=w485:refnum<queue>)  [unwired: 6 in]
        n161 = case shown="True" w488 {
          tunnel: w487 -> [w498 w502]
          tunnel: w485 -> [_ w501]
          tunnel: [w498 w499] -> w496
          frame False {
          }
          frame True {
            n162 = call <userlib>:"Enqueue Message (Single).vi"("error in (no error)"=w502, "Message"="Start", "Message Queue"=w501) -> ("error out"=w499:errorcluster)  [unwired: 7 in, 1 out]
          }
        }
        n163 = call <userlib>:"Enqueue Message (Single).vi"("error in (no error)"=w496, "Message"="Start", "Message Queue"=w495) -> ("error out"=w478:errorcluster)  [unwired: 7 in, 1 out]
        n164 = Unbundle By Name(w489) -> ("Clone"=w491:bool)
        n165 = Variant To Data(error in=w478, type=T10 {"VISA Resource"="", "Address"=0} ("Connection Info"), Variant=w477) -> (data=w479:T10, error out=w475:errorcluster)
        n166 = call "Serialize Connection Info.vi"("error in (no error)"=w475, "Connection Info"=w479) -> ("error out 2"=w480:errorcluster, "Serialized Connection Info"=w481:string)  [unwired: 8 in]
        n167 = call <userlib>:"Enqueue Message (Single).vi"("error in (no error)"=w480, "Message Data"=w481, "Message"=w476, "Message Queue"=w494) -> ("error out"=w492:errorcluster)  [unwired: 6 in, 1 out]
        n168 = case shown="True" w491 {
          tunnel: w492 -> [w506 w507]
          tunnel: [w505 w507] -> w490
          tunnel: w493 -> [w504 _]
          frame False {
            # "Show the Front Panel automatically on startup"
            n169 = call <userlib>:"Enqueue Message (Single).vi"("error in (no error)"=w506, "Message"="Show", "Message Queue"=w504) -> ("error out"=w505:errorcluster)  [unwired: 7 in, 1 out]
          }
          frame True {
            # "Reentrant clone. It is the responsibility of the RCM to send \"Show\" if the plugin UI is desired."
          }
        }
      }
      frame "Invalid Connection Info" {
        # "On invalid connection info, ask the user to try to fix it."
        n170 = call <userlib>:"Enqueue Message (Single).vi"("error in (no error)"=w512, "Message Data"=w508, "Message"="Get Connection Info", "Message Queue"=w510) -> ("error out"=w511:errorcluster)  [unwired: 6 in, 1 out]
      }
      frame "Start Logging", "Stop Logging" {
        # "Extract if this is the start or stop command"
        # "Forward the message to start or stop logging."
        n171 = Scan From String(format string="%s Logging", input string=w515, error in=w517) -> (error out=w516:errorcluster, output 1=w514:string)  [unwired: 2 in, 2 out]
        n172 = call <userlib>:"Enqueue Message (Single).vi"("Priority Message? (F)"=TRUE, "error in (no error)"=w516, "Message"=w514, "Message Queue"=w520) -> ("error out"=w521:errorcluster)  [unwired: 6 in, 1 out]
        n173 = Merge Errors(w521) -> (w522:errorcluster)
      }
      frame "Open Settings" {
        # "Message to open the settings dialog."
        n174 = call <userlib>:"Enqueue Message (Single).vi"("error in (no error)"=w528, "Message Data"=w526, "Message"=w525, "Message Queue"=w524) -> ("error out"=w527:errorcluster)  [unwired: 6 in, 1 out]
        n175 = Merge Errors(w527) -> (w529:errorcluster)
      }
      frame "Open Calibrate Menu" {
        # "Message to open the settings dialog."
        n176 = call <userlib>:"Enqueue Message (Single).vi"("error in (no error)"=w535, "Message Data"=w533, "Message"=w532, "Message Queue"=w531) -> ("error out"=w534:errorcluster)  [unwired: 6 in, 1 out]
        n177 = Merge Errors(w534) -> (w536:errorcluster)
      }
      frame "Acquisition Config", "Instrument Config", "Logging Config" {
        # "#todo: This may get sent to RCM later"
        # "A process loop reporting its public config values."
        n178 = call <userlib>:"Enqueue Message (Single).vi"("error in (no error)"=w542, "Message Data"=w540, "Message"=w539, "Message Queue"=w538) -> ("error out"=w541:errorcluster)  [unwired: 6 in, 1 out]
        n179 = Merge Errors(w541) -> (w543:errorcluster)
      }
      frame "New Acquisition Config", "New Instrument Config", "New Logging Config" {
        # "Send new settings to the corresponding process loop."
        n180 = Scan From String(format string="New %s Config", input string=w552, error in=w554) -> (error out=w547:errorcluster, output 1=w551:string)  [unwired: 2 in, 2 out]
        n181 = call <userlib>:"Get Queue by Name.vi"("error in (no error)"=w547, "Queue Name"=w551, "Message Queues in"=w545) -> ("error out"=w546:errorcluster, "Queue out"=w548:refnum<queue>)  [unwired: 7 in]
        n182 = call <userlib>:"Enqueue Message (Single).vi"("error in (no error)"=w546, "Message Data"=w550, "Message"=w552, "Message Queue"=w548) -> ("error out"=w549:errorcluster)  [unwired: 6 in, 1 out]
        n183 = Merge Errors(w549) -> (w555:errorcluster)
      }
      frame "Set Entry Names", "Set Log Directory", "Set Log File Delimiter", "Set Log File Prefix", "Set Log on Run" {
        # "Pass on message to set a logging config value to the Logging Loop."
        n184 = call <userlib>:"Enqueue Message (Single).vi"("error in (no error)"=w561, "Message Data"=w558, "Message"=w557, "Message Queue"=w559) -> ("error out"=w560:errorcluster)  [unwired: 6 in, 1 out]
        n185 = Merge Errors(w560) -> (w562:errorcluster)
      }
      frame "Set Acquisition Messages" {
        # "Pass on message to set the acquisition messages."
        n186 = call <userlib>:"Enqueue Message (Single).vi"("error in (no error)"=w568, "Message Data"=w566, "Message"=w565, "Message Queue"=w564) -> ("error out"=w567:errorcluster)  [unwired: 6 in, 1 out]
        n187 = Merge Errors(w567) -> (w569:errorcluster)
      }
      frame "Logging Started", "Logging Stopped" {
        # "Pass on Logging status message to RCM and UI."
        n188 = Build Array(w572, w573) -> (w571:refnum<queue>[])
        n189 = for {
          tunnel: w575 -> [w582]
          tunnel: w574 -> [w581]
          shift-right: [w583] -> w576
          shift-left: w577 -> [w584]
          tunnel: w571 -> [w580] mode=indexing
          n190 = call <userlib>:"Enqueue Message (Single).vi"("error in (no error)"=w584, "Message Data"=w582, "Message"=w581, "Message Queue"=w580) -> ("error out"=w583:errorcluster)  [unwired: 6 in, 1 out]
        }
        n191 = Merge Errors(w576) -> (w578:errorcluster)
      }
      frame "Change Refresh" {
        # "Change the sampling rate of the instrument. Default value is the default set on the front panel control."
        n192 = Build Array(w586) -> (w585:refnum<queue>[])
        n193 = for {
          tunnel: w588 -> [w595]
          tunnel: w587 -> [w594]
          tunnel: w585 -> [w593] mode=indexing
          shift-right: [w596] -> w589
          shift-left: w592 -> [w597]
          n194 = call <userlib>:"Enqueue Message (Single).vi"("error in (no error)"=w597, "Message Data"=w594, "Message"=w595, "Message Queue"=w593) -> ("error out"=w596:errorcluster)  [unwired: 6 in, 1 out]
        }
        n195 = Merge Errors(w589) -> (w590:errorcluster)
      }
      frame "Calibrate High", "Calibrate Low", "Calibrate Mid", "Clear Calibration", "Enter CONFIG", "Exit CONFIG", "Reset to Factory Default", "Restart", "Save Calibration", "Set Address", "Set Compensation Temperature", "Start Instrument", "Stop Instrument" {
        # "Pass action message to Instrument Manager Loop."
        n196 = call <userlib>:"Enqueue Message (Single).vi"("error in (no error)"=w602, "Message Data"=w600, "Message"=w599, "Message Queue"=w598) -> ("error out"=w601:errorcluster)  [unwired: 6 in, 1 out]
        n197 = Merge Errors(w601) -> (w603:errorcluster)
      }
      frame "Instrument Started", "Instrument Stopped" {
        # "Build an array of all processes that will receive this message"
        # "Notify processes of update"
        # "Notify processes of the instrument run state change."
        n198 = Build Array(w605, w612, w607, w606) -> (w613:refnum<queue>[])
        n199 = for {
          tunnel: w613 -> [w617] mode=indexing
          tunnel: w610 -> [w619]
          tunnel: w611 -> [w618]
          shift-right: [w616] -> w609
          shift-left: _ -> [w614]
          n200 = call <userlib>:"Enqueue Message (Single).vi"("Message Data"=w618, "Message"=w619, "Message Queue"=w617) -> ("error out"=w615:errorcluster)  [unwired: 7 in, 1 out]
          n201 = Merge Errors(w615, w614) -> (w616:errorcluster)
        }
      }
      frame "Report" {
        # "Convert to RCM"
        # "Send instrument state notification"
        # "Notify processes that the instrument stopped running."
        n202 = Variant To Data(error in=w629, type=T12 {"Connection Info"={"VISA Resource"="", "Address"=0}, "Running"=FALSE, "Running Since"=timestamp(0 s since 1904-01-01), "Instrument State"={"pH"=0.0, "Temperature (C)"=0.0, "Device"="", "Firmware Version"="", "Error Status"=FALSE, "Error Code"=0, "Error Source"=""}} ("Instrument State"), Variant=w623) -> (data=w620:T12, error out=w628:errorcluster)
        n203 = Unbundle By Name(w624) -> ("Remote"=w636:refnum<queue>)
        n204 = call "To JSON Text.vim"("Anything"=w620) -> ("<JSON>"=w622:string)  [unwired: 9 in, 1 out]
        n205 = call "Convert to Remote Instrument State.vi"("Internal Instrument State in"=w620) -> ("Remote Instrument State out"=w621:variant)  [unwired: 9 in, 1 out]
        n206 = Enqueue Element(queue=w630, element=w622, error in (no error)=w628) -> (error out=w625:errorcluster)  [unwired: 1 in, 2 out]
        n207 = Send Notification(notification=w620, notifier=w632, error in (no error)=w628) -> (error out=w626:errorcluster)  [unwired: 1 out]
        n208 = call <userlib>:"Enqueue Message (Single).vi"("error in (no error)"=w628, "Message Data"=w621, "Message"=w635, "Message Queue"=w636) -> ("error out"=w634:errorcluster)  [unwired: 6 in, 1 out]
        n209 = Merge Errors(w625, w626, w634) -> (w627:errorcluster)
      }
      frame "Valid Port Mappings" {
        # "Notify processes that the instrument stopped running."
      }
    }
    n210 = call "Error Handler - System Control Loop.vi"("error in (no error)"=w317, "Message Queue"=w319) -> ("dup error in"=w318:errorcluster)  [unwired: 8 in, 1 out]
  }
  n211 = call "Instrument Manager Loop.vi"("System Control"=w4, "Instrument Manager"=w35) -> ("error out"=w20:errorcluster)  [unwired: 9 in]
  n212 = call <userlib>:"Logging Message Loop.vi"("System Control"=w4, "Data Queue"=w1, "Logging"=w34) -> ("error out"=w19:errorcluster)  [unwired: 8 in]
  n213 = call <userlib>:"Acquisition Message Loop.vi"("System Control"=w4, "Instrument Manager"=w35, "Acquisition"=w33) -> ("error out"=w18:errorcluster)  [unwired: 8 in]
  n214 = call <userlib>:"Remote Connection Manager Loop.vi"("System Control"=w4, "IsCloneVI (false)"=w23, "Remote"=w32) -> ("error out"=w8:errorcluster)  [unwired: 8 in]
  n215 = Unregister For Events(event registration refnum=w26) -> (error out=w21:errorcluster)  [unwired: 1 in]
  n216 = Merge Errors(w30, w22, w21, w20, w19, w18, w8) -> (w16:errorcluster)
  n217 = call <vilib>:"Simple Error Handler.vi"("error in (no error)"=w16) -> ()  [unwired: 4 in, 5 out]
  n218 = Cluster To Array(cluster=w7) -> (array=w15:refnum<queue>[])
  n219 = for {
    shift-right: [w640] -> w14
    shift-left: w16 -> [w641]
    tunnel: w15 -> [w642] mode=indexing
    n220 = Release Queue(queue=w642, force destroy? (F)=TRUE, error in (no error)=w641) -> (error out=w640:errorcluster)  [unwired: 2 out]
  }
  n221 = call <userlib>:"Destroy User Event - Stop.vi"("error in (no error)"=w14, "User Event - Stop"=w25) -> ("error out"=w27:errorcluster)  [unwired: 9 in]
  n222 = disable-structure shown="RUN_TIME_ENGINE==True" {
    disable-tunnel: w27 -> [_ _]
    frame condition #0 (active) {
    }
    frame condition #1 {
      # "Call Quit LabVIEW if running as a built application."
      n223 = Quit LabVIEW() -> ()  [unwired: 1 in]
    }
  }
